vi "Write Data Rate.vi"(8 "error in (no error)":errorcluster, 10 "Rate":dbl, 11 "Daqmx Module configuration in":refnum<class "Daqmx Module configuration.lvclass">) -> (0 "error out":errorcluster, 3 "Daqmx Module configuration out":refnum<class "Daqmx Module configuration.lvclass">)   [LabVIEW 2014, in "DAQmx Module Configuration.lvclass"]
uses:
  Daqmx Module configuration.lvclass
  Daqmx Module configuration.lvclass/Daqmx Module configuration.ctl
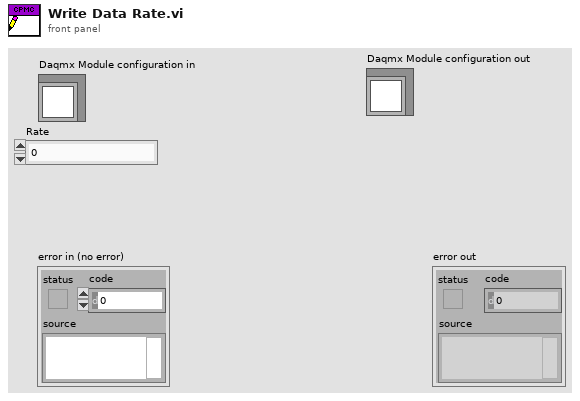
[diagram p1: front panel]
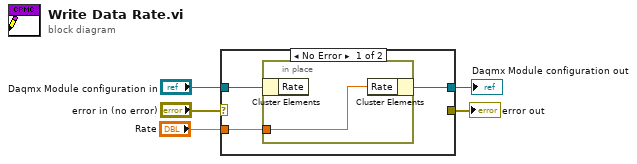
[diagram p0: block diagram]
diagram:
  n1 = case shown="No Error" "error in (no error)" {
    selector: "error in (no error)" -> [_ w11]
    tunnel: [_ w11] -> w4
    tunnel: "Daqmx Module configuration in" -> [w7 w10]
    tunnel: "Rate" -> [w8 _]
    tunnel: [w6 w10] -> w1
    frame No Error {
      n2 = in-place {
        in-place-border: w8 -> [w9]
        n3 = in-place-cluster #1(w7) -> ()  [unwired: 1 out]
        n4 = in-place-cluster #1("Rate"=w9) -> (w6:refnum<class "Daqmx Module configuration.lvclass">)
      }
    }
    frame Error {
    }
  }
  "error out" <- w4
  "Daqmx Module configuration out" <- w1
